vi "Unpack AI Data.vi"(10 "Packet AI Data":u8[](array[numeric])) -> (0 "AI3":dbl, 1 "AI2":dbl, 2 "AI1":dbl, 3 "AI0":dbl)   [LabVIEW 2011, in "LabVIEW Interface for ChipKit.lvlib"]
uses:
  LabVIEW Interface for ChipKit.lvlib
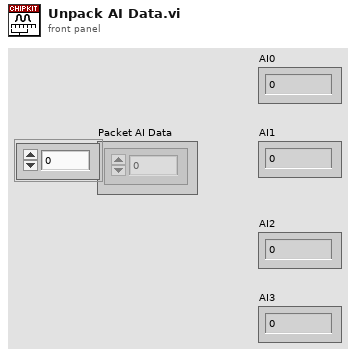
[diagram p1: front panel]
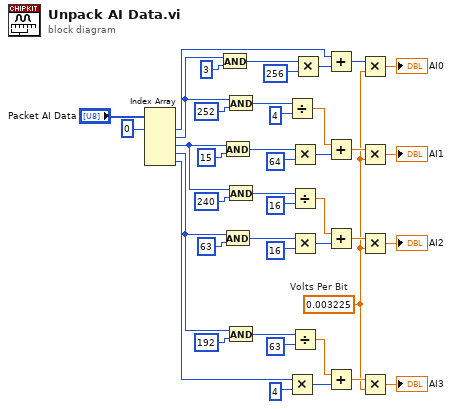
[diagram p0: block diagram]
diagram:
  w1 = 0.003225  # Volts Per Bit
  n1 = Index Array(array="Packet AI Data", index #1=0 ("index")) -> (element #1=w8:u8, element #2=w10:u8, element #3=w20:u8, element #4=w40:u8, element #5=w42:u8)  [unwired: 4 in]
  n2 = And(x=w10, y=u8 3) -> (x .and. y?=w5:u8)
  n3 = And(x=w20, y=u8 15) -> (x .and. y?=w18:u8)
  n4 = And(x=w40, y=u8 63) -> (x .and. y?=w25:u8)
  n5 = And(x=w10, y=u8 252) -> (x .and. y?=w12:u8)
  n6 = And(x=w20, y=u8 240) -> (x .and. y?=w22:u8)
  n7 = And(x=w40, y=u8 192) -> (x .and. y?=w38:u8)
  n8 = Divide(x=w12, y=u8 4) -> (x/y=w19:dbl)
  n9 = Multiply(x=w42, y=u16 4) -> (x*y=w33:u16)
  n10 = Multiply(x=w18, y=u16 64) -> (x*y=w16:u16)
  n11 = Divide(x=w22, y=u8 16) -> (x/y=w24:dbl)
  n12 = Multiply(x=w25, y=u16 16) -> (x*y=w29:u16)
  n13 = Divide(x=w38, y=u8 63) -> (x/y=w36:dbl)
  n14 = Multiply(x=w5, y=u16 256) -> (x*y=w7:u16)
  n15 = Add(x=w8, y=w7) -> (x+y=w9:u16)
  n16 = Add(x=w19, y=w16) -> (x+y=w15:dbl)
  n17 = Add(x=w24, y=w29) -> (x+y=w23:dbl)
  n18 = Add(x=w36, y=w33) -> (x+y=w37:dbl)
  n19 = Multiply(x=w9, y=w1) -> (x*y=→"AI0":dbl)
  n20 = Multiply(x=w15, y=w1) -> (x*y=→"AI1":dbl)
  n21 = Multiply(x=w23, y=w1) -> (x*y=→"AI2":dbl)
  n22 = Multiply(x=w37, y=w1) -> (x*y=→"AI3":dbl)
